vi "verify module configuration.vi"(8 "error in":errorcluster, 11 "module editor node in":refnum<class "module editor node.lvclass">) -> (0 "error out":errorcluster, 3 "module editor node out":refnum<class "module editor node.lvclass">)   [LabVIEW 2013, in "PL Framework Configuration Tool.lvlib" / "module editor node.lvclass"]
uses:
  module editor node.lvclass
  module editor node.lvclass/module editor node.ctl
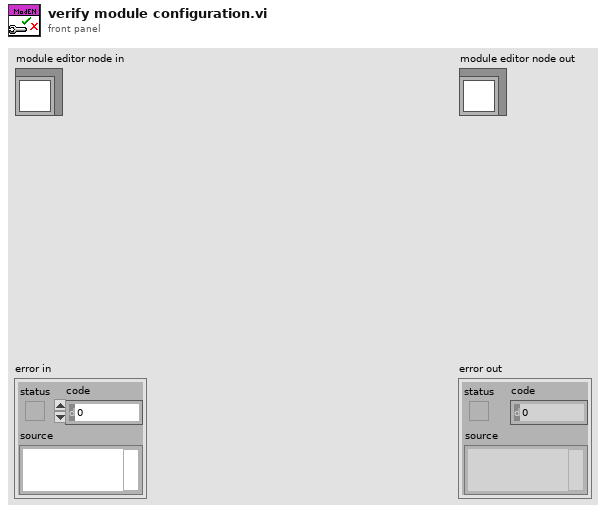
[diagram p1: front panel]
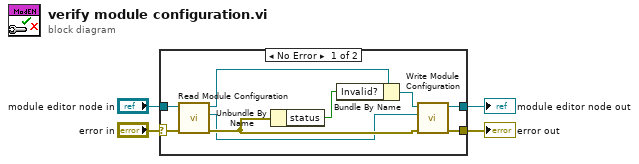
[diagram p0: block diagram]
diagram:
  n1 = case shown="No Error" "error in" {
    selector: "error in" -> [w5 w15]
    tunnel: "module editor node in" -> [w7 w14]
    tunnel: [w10 w15] -> w3
    tunnel: [w11 w14] -> w2
    frame No Error {
      n2 = call "Read Module Configuration.vi"("error in"=w5, "Module Editor Node in"=w7) -> ("error out"=w9:errorcluster, "module configuration"=w8:refnum<class "TBM module configuration.lvclass">, "Module Editor Node out"=w6:refnum<class "module editor node.lvclass">)  [unwired: 7 in]
      n3 = Unbundle By Name(w9) -> ("status"=w13:bool)
      n4 = Bundle By Name(cluster=w6, "Invalid?"=w13) -> (w12:refnum<class "module editor node.lvclass">)
      n5 = call "Write Module Configuration.vi"("error in"=w9, "module configuration"=w8, "Module Editor Node in"=w12) -> ("error out"=w10:errorcluster, "Module Editor Node out"=w11:refnum<class "module editor node.lvclass">)  [unwired: 7 in]
    }
    frame Error {
    }
  }
  "error out" <- w3
  "module editor node out" <- w2
